vi "ClosePMT.vi"(11 "Handle":i32) -> (2 "Return":i32, 3 "Handle out":i32)   [LabVIEW 2022 SP3]
doc: "BOOL H11890API __stdcall H11890Close(HANDLE hDeviceHandle);"
uses:
  H11890api.dll
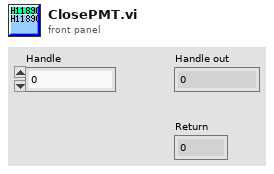
[diagram p1: front panel]
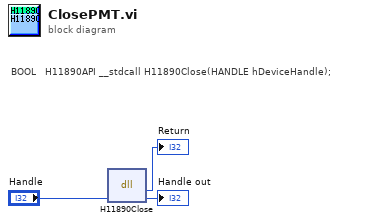
[diagram p0: block diagram]
diagram:
  # "BOOL\t\t\tH11890API __stdcall H11890Close(HANDLE hDeviceHandle);"
  n1 = dll-call lib="C:/Users/Public/OneDrive/Desktop/PMT_Project_folder/PMT_VIs/H11890api.dll" fn="H11890Close"("Handle"="Handle") -> ("Return"=→"Return":i32, "Handle"=→"Handle out":i32)  [unwired: 3 in, 2 out]
